vi "Nested Exist.vi"(11 "jettl Queue Actor in":refnum<class "jettl Queue Actor.lvclass">) -> (2 "Nested Exist?":bool)   [LabVIEW 2021, in "jettl.lvlib" / "jettl Queue Actor.lvlib" / "jettl Queue Actor.lvclass"]
uses:
  jettl Queue Actor.lvclass
  jettl Queue Actor.lvclass/jettl Queue Actor.ctl
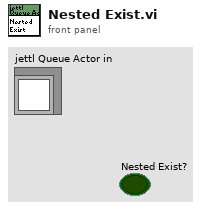
[diagram p1: front panel]
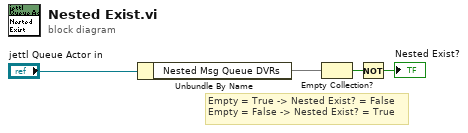
[diagram p0: block diagram]
diagram:
  # "Empty = True -> Nested Exist? = False\nEmpty = False -> Nested Exist? = True"
  n1 = Unbundle By Name("jettl Queue Actor in") -> ("Nested Msg Queue DVRs"=w2:map{string, refnum<data-value>})
  n2 = Empty Collection?(1:w2) -> (0:w1:bool)
  n3 = Not(x=w1) -> (.not. x?=→"Nested Exist?":bool)
